vi "Execute.vi"(8 "error in (no error)":errorcluster, 10 "Abstract Consumer in":refnum<class "Abstract Consumer.lvclass">, 11 "Count Request Message in":refnum<class "Count Request Message.lvclass">) -> (0 "error out":errorcluster, 1 "Abstract Response out":refnum<class "Abstract Response Message.lvclass">, 2 "Abstract Consumer out":refnum<class "Abstract Consumer.lvclass">, 3 "Count Request Message out":refnum<class "Count Request Message.lvclass">, 4 "Stop?":bool)   [LabVIEW 2027, in "Count Request Message.lvclass"]
uses:
  Count Request Message.lvclass
  Consumer/Abstract Consumer/Abstract Consumer.lvclass
  Message/Abstract Response Message/Abstract Response Message.lvclass
  Count Response Message/Count Response Message.lvclass
  Message List Action.ctl
  Count Request Message.lvclass/Count Request Message.ctl
  Count Response Message/Count Response Message.lvclass/Count Response Message.ctl
  Count Response Message/Write Count.vi
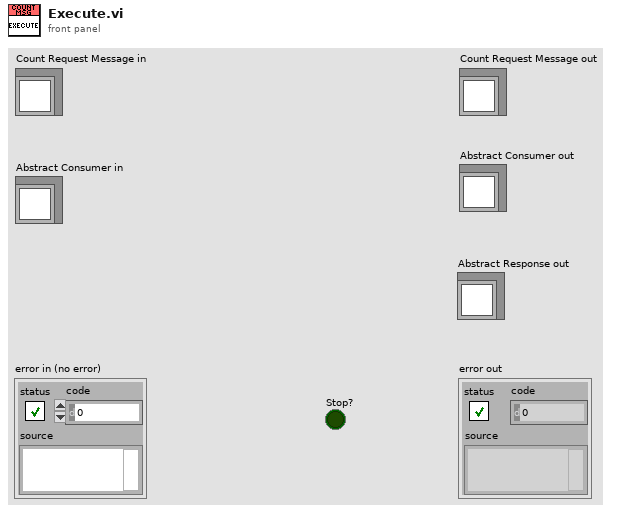
[diagram p1: front panel]
types:
  T1 = typedef "Message List Action.ctl" = enum16{"Get", "Add", "Reset"}
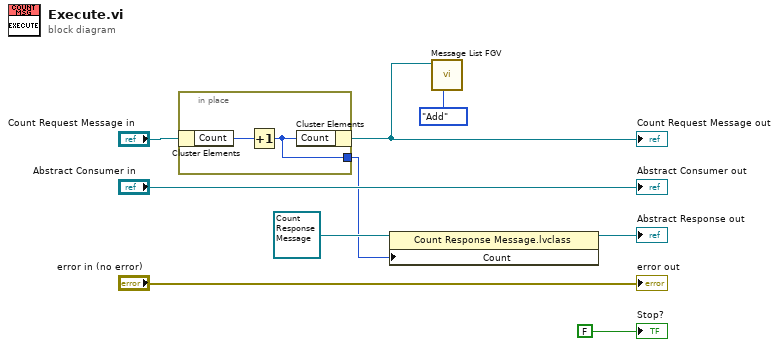
[diagram p0: block diagram]
diagram:
  n1 = in-place {
    in-place-border: [w10] -> w3
    n2 = in-place-cluster #1("Count Request Message in") -> ("Count"=w11:u32)
    n3 = Increment(x=w11) -> (x+1=w10:u32)
    n4 = in-place-cluster #1("Count"=w10) -> (w2:refnum<class "Count Request Message.lvclass">)
  }
  "Count Request Message out" <- w2
  n5 = property class="Count Response Message.lvclass"(reference=refnum<class "Count Response Message.lvclass"> refnum ("Count Response Message.lvclass"), "Count"=w3) -> (reference out=→"Abstract Response out":refnum<class "Count Response Message.lvclass">)  [unwired: 1 in, 1 out]
  n6 = call "Message List FGV.vi"("Action (Get)"=Message_List_Action."Add", "Message Object"=w2) -> ()  [unwired: 8 in, 2 out]
  "error out" <- "error in (no error)"
  "Abstract Consumer out" <- "Abstract Consumer in"
  "Stop?" <- FALSE ("Stop?")
